vi "Visualization Module.vi"(7 "XY graph buffer size":i32=1000, 8 "error in":errorcluster, 9 "Vector Space Setup":enum16{"Coordinate Space", "Single Axes"}(ring), 10 "Coordinate Space":refnum<k21>="Coordinate Space 1", 11 "Motion Resources":refnum<k21>[](array[refnum])=["Axis 1", "Axis 2", "Axis 3", "Axis 4"]) -> (0 "error out":errorcluster)   [LabVIEW 2014]
uses:
  Globals/Global Stop.vi
  <vilib>/Motion/Express/_s/nimc.ex.read.readTrajectoryData.coordinate.vi
  <vilib>/Motion/Express/_s/nimc.ex.read.readTrajectoryData.axis.vi
  <vilib>/Motion/BlockNode/FB.NIMotion.xnode
panel:
  in  "Tab Control":T1(tab)
  out "XY Plot":cluster{dbl[], dbl[]}(graph)
  out "Axis Positions":T2(graph)={"commanded pos.[] out[0]"=37.92979683924918, "commanded pos.[] out[1]"=28.694528189915523, "commanded pos.[] out[2]"=-0.5077, "commanded pos.[] out[3]"=0.0}
  out "Axis Velocities":T3(graph)={"velocity"=5.4381925081040325, "velocity"=15.450685803910837, "velocity"=0.0, "velocity"=0.0}
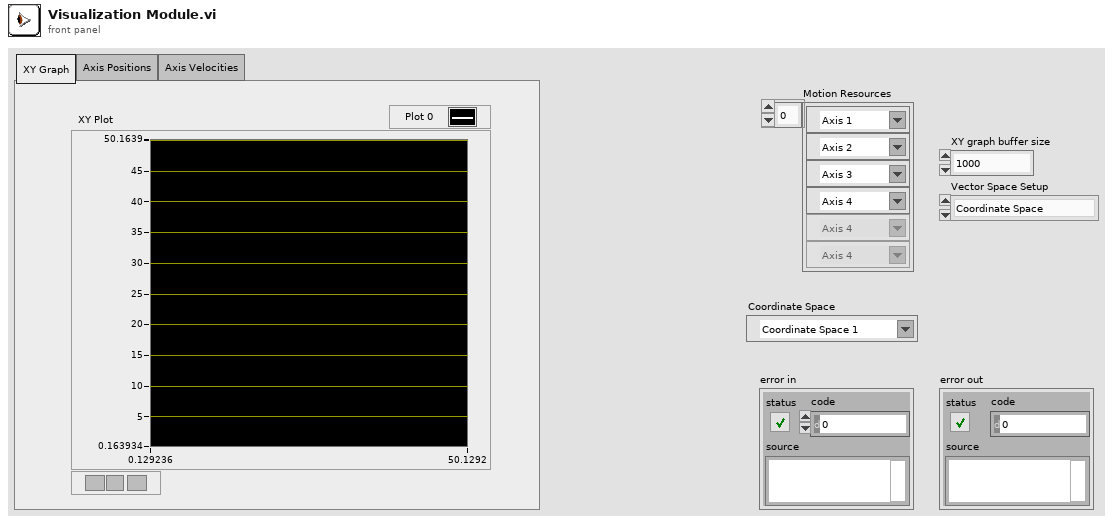
[diagram p1: front panel]
types:
  T1 = enum32{"XY Graph", "Axis Positions", "Axis Velocities"}
  T2 = cluster{"commanded pos.[] out[0]":dbl, "commanded pos.[] out[1]":dbl, "commanded pos.[] out[2]":dbl, "commanded pos.[] out[3]":dbl}
  T3 = cluster{"velocity":dbl, "velocity":dbl, "velocity":dbl, "velocity":dbl}
  T4 = cluster{"[0]":dbl, "[1]":dbl, "[2]":dbl, "[3]":dbl}
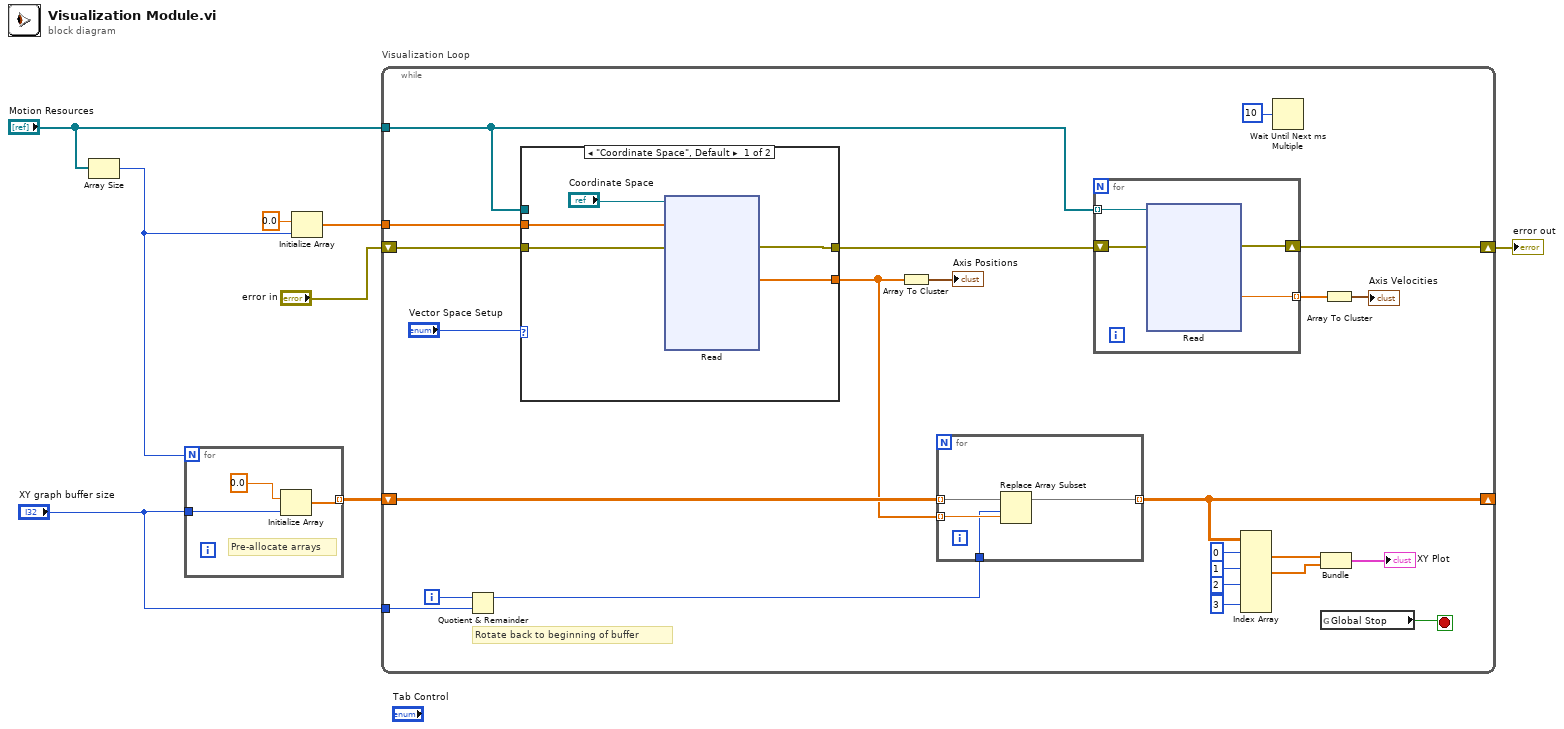
[diagram p0: block diagram]
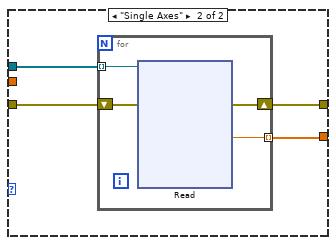
[diagram p2: hidden frame]
diagram:
  n1 = Array Size(array="Motion Resources") -> (size(s)=w3:i32)
  n2 = for {
    N: w3 -> [_]
    tunnel: [w10] -> w2 mode=indexing
    tunnel: "XY graph buffer size" -> [w9]
    # "Pre-allocate arrays"
    n3 = Initialize Array(0.0 ("element"), w9) -> (w10:dbl[])
  }
  n4 = Initialize Array(0.0 ("element"), w3) -> (w7:dbl[])
  n5 = while "Visualization Loop" {
    shift-right: [w28] -> w6
    shift-left: "error in" -> [w31]
    tunnel: "XY graph buffer size" -> [w34]
    tunnel: w7 -> [w29]
    tunnel: "Motion Resources" -> [w16]
    shift-right: [w15] -> _
    shift-left: w2 -> [w26]
    i -> [w33]
    stop <- w27 stop-if-true
    # "Rotate back to beginning of buffer"
    n6 = Quotient & Remainder(x=w33, y=w34) -> (x-y*floor(x/y)=w24:i32)  [unwired: 1 out]
    n7 = case shown="\"Coordinate Space\", Default" "Vector Space Setup" {
      tunnel: w31 -> [w40 w52]
      tunnel: [w39 w51] -> w30
      tunnel: w29 -> [w38 _]
      tunnel: [w36 w50] -> w25
      tunnel: w16 -> [_ w53]
      frame "Coordinate Space", Default {
        n8 = xnode ("Read")("resource"="Coordinate Space", "commanded pos.[]"=w38, "error in"=w40) -> ("commanded pos.[] out"=w36:dbl[], "error out"=w39:errorcluster)  [unwired: 4 out]
      }
      frame "Single Axes" {
        n9 = for {
          tunnel: w53 -> [w57] mode=indexing
          shift-right: [w55] -> w51
          shift-left: w52 -> [w56]
          tunnel: [w54] -> w50 mode=indexing
          n10 = xnode ("Read")("resource"=w57, "error in"=w56) -> ("commanded position"=w54:dbl, "error out"=w55:errorcluster)  [unwired: 3 out]
        }
      }
    }
    n11 = Array To Cluster(array=w25) -> (cluster=→"Axis Positions":T2)
    n12 = for {
      tunnel: w26 -> [w68] mode=indexing
      tunnel: w25 -> [w67] mode=indexing
      tunnel: w24 -> [w66]
      tunnel: [w65] -> w15 mode=indexing
      n13 = Replace Array Subset(array=w68, new element=w67, index=w66) -> (w65:dbl[])
    }
    n14 = for {
      tunnel: w16 -> [w72] mode=indexing
      tunnel: [w69] -> w14 mode=indexing
      shift-right: [w70] -> w28
      shift-left: w30 -> [w71]
      n15 = xnode ("Read")("resource"=w72, "error in"=w71) -> ("commanded vel."=w69:dbl, "error out"=w70:errorcluster)  [unwired: 3 out]
    }
    n16 = Index Array(array=w15, index (row) #1=0 ("index (row)"), index (row) #2=1 ("index (row)"), index (row) #3=2 ("index (row)"), index (row) #4=3 ("index (row)")) -> (element #1=w18:dbl[], element #2=w20:dbl[])  [unwired: 4 in, 2 out]
    n17 = Wait Until Next ms Multiple(millisecond multiple=u32 10) -> ()  [unwired: 1 out]
    n18 = Bundle(w18, w20) -> (→"XY Plot":cluster{dbl[], dbl[]})  [unwired: 1 in]
    n19 = global read "Global Stop.vi" "Global Stop"() -> (w27:bool)
    n20 = Array To Cluster(array=w14) -> (cluster=→"Axis Velocities":T4)
  }
  "error out" <- w6
